vi "CLD3 FGV Timer no pause solution.vi"(8 "error in (no error)":errorcluster, 10 "Wait":dbl, 11 "Timer Task":T1) -> (0 "error out":errorcluster, 2 "Time elapsed?":bool, 3 "Elapsed Time":dbl)   [LabVIEW 2009]
doc: "CLD 3 challenge Exercise\n\nSimple elapsed time timer. Uses time stamp comparison to get difference in seconds."
uses:
  CLD3 Timer Mode.ctl
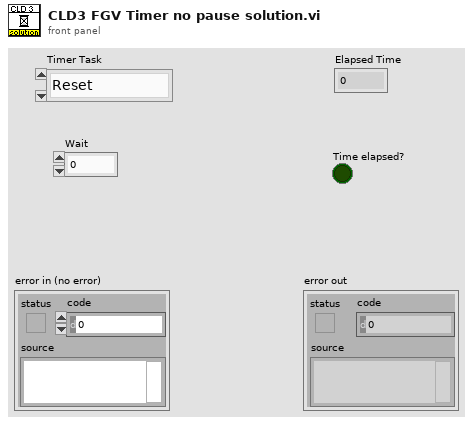
[diagram p1: front panel]
types:
  T1 = typedef "CLD3 Timer Mode.ctl" = enum16{"Reset", "Elapsed"}
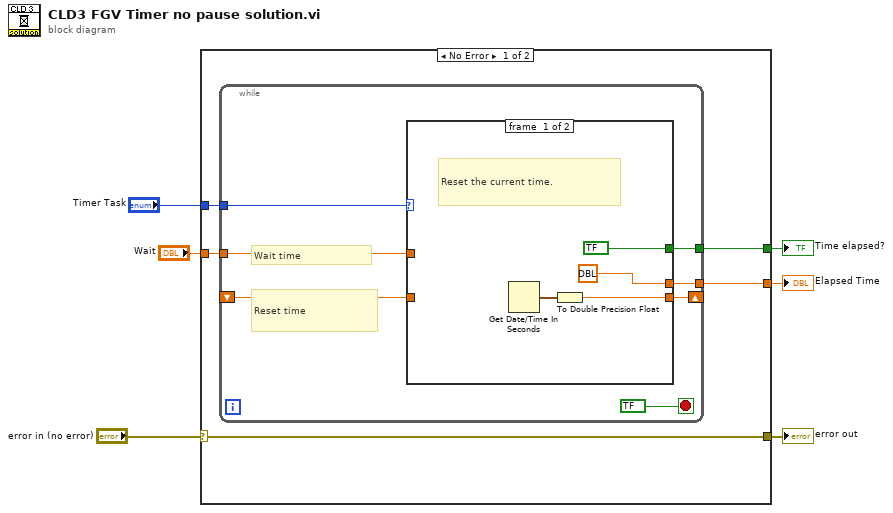
[diagram p0: block diagram]
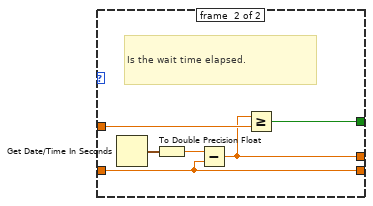
[diagram p2: hidden frame]
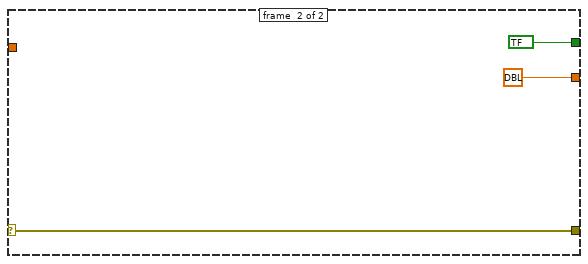
[diagram p3: hidden frame]
diagram:
  n1 = case shown="No Error" "error in (no error)" {
    selector: "error in (no error)" -> [w8 w31]
    tunnel: "Timer Task" -> [w11 _]
    tunnel: "Wait" -> [w10 _]
    tunnel: [w9 bool ?] -> w5
    tunnel: [w8 w31] -> w3
    tunnel: [w7 dbl ?] -> w2
    frame #0 {
      n2 = while {
        tunnel: w11 -> [w17]
        shift-right: [w16] -> _
        shift-left: _ -> [w15]
        tunnel: w10 -> [w14]
        tunnel: [w13] -> w9
        tunnel: [w12] -> w7
        stop <- bool ? stop-if-true
        # "Reset time"
        # "Wait time"
        n3 = case shown="\"Elapsed\"" w17 {
          tunnel: [w21 w23] -> w16
          tunnel: w15 -> [_ w23]
          tunnel: w14 -> [_ w27]
          tunnel: [bool ? w26] -> w13
          tunnel: [dbl ? w25] -> w12
          frame #0 {
            # "Reset the current time."
            n4 = Get Date/Time In Seconds() -> (seconds since 1Jan1904=w22:timestamp)
            n5 = To Double Precision Float(number=w22) -> (double precision float=w21:dbl)
          }
          frame #1 {
            # "Is the wait time elapsed."
            n6 = Get Date/Time In Seconds() -> (seconds since 1Jan1904=w28:timestamp)
            n7 = To Double Precision Float(number=w28) -> (double precision float=w24:dbl)
            n8 = Subtract(x=w24, y=w23) -> (x-y=w25:dbl)
            n9 = Greater Or Equal?(x=w25, y=w27) -> (x >= y?=w26:bool)
          }
        }
      }
    }
    frame #1 {
    }
  }
  "Time elapsed?" <- w5
  "error out" <- w3
  "Elapsed Time" <- w2
